vi "FXP NILIA_Shift_Arith.vi"(9 "dec":i32, 11 "x":i64) -> (3 "y":i64)   [LabVIEW 2012]
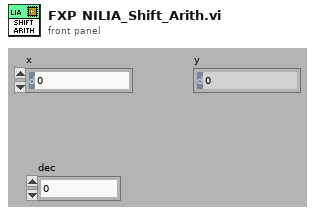
[diagram p1: front panel]
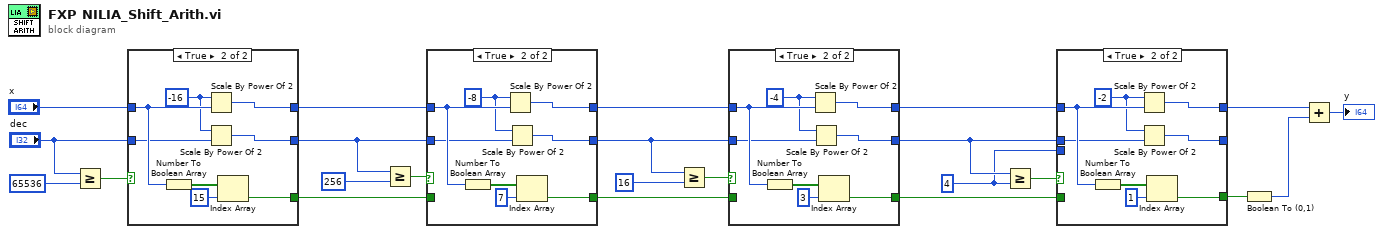
[diagram p0: block diagram]
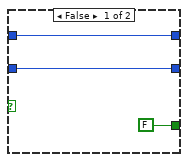
[diagram p5: hidden frame]
diagram:
  w8 = 4
  n1 = Greater Or Equal?(x="dec", y=65536) -> (x >= y?=w23:bool)
  n2 = case shown="True" w23 {
    tunnel: "x" -> [w26 w33]
    tunnel: [w26 w34] -> w16
    tunnel: "dec" -> [w25 w29]
    tunnel: [w25 w27] -> w19
    tunnel: [FALSE w30] -> w7
    frame False {
    }
    frame True {
      w28 = -16
      n3 = Number To Boolean Array(number=w33) -> (Boolean array=w32:bool[])
      n4 = Scale By Power Of 2(n=w28, x=w33) -> (x*2^n=w34:i64)
      n5 = Scale By Power Of 2(n=w28, x=w29) -> (x*2^n=w27:i32)
      n6 = Index Array(array=w32, index=15) -> (element=w30:bool)
    }
  }
  n7 = Greater Or Equal?(x=w19, y=256) -> (x >= y?=w18:bool)
  n8 = case shown="True" w18 {
    tunnel: w16 -> [w37 w44]
    tunnel: [w37 w45] -> w15
    tunnel: w19 -> [w36 w40]
    tunnel: [w36 w39] -> w13
    tunnel: w7 -> [w35 _]
    tunnel: [w35 w41] -> w6
    frame False {
    }
    frame True {
      w38 = -8
      n9 = Number To Boolean Array(number=w44) -> (Boolean array=w43:bool[])
      n10 = Scale By Power Of 2(n=w38, x=w44) -> (x*2^n=w45:i64)
      n11 = Scale By Power Of 2(n=w38, x=w40) -> (x*2^n=w39:i32)
      n12 = Index Array(array=w43, index=7) -> (element=w41:bool)
    }
  }
  n13 = Greater Or Equal?(x=w13, y=16) -> (x >= y?=w14:bool)
  n14 = case shown="True" w14 {
    tunnel: w15 -> [w48 w55]
    tunnel: [w48 w56] -> w11
    tunnel: w13 -> [w47 w51]
    tunnel: [w47 w50] -> w10
    tunnel: [w46 w52] -> w5
    tunnel: w6 -> [w46 _]
    frame False {
    }
    frame True {
      w49 = -4
      n15 = Number To Boolean Array(number=w55) -> (Boolean array=w54:bool[])
      n16 = Scale By Power Of 2(n=w49, x=w55) -> (x*2^n=w56:i64)
      n17 = Scale By Power Of 2(n=w49, x=w51) -> (x*2^n=w50:i32)
      n18 = Index Array(array=w54, index=3) -> (element=w52:bool)
    }
  }
  n19 = Greater Or Equal?(x=w10, y=w8) -> (x >= y?=w9:bool)
  n20 = case shown="True" w9 {
    tunnel: w11 -> [w59 w66]
    tunnel: [w59 w67] -> w4
    tunnel: w10 -> [w58 w62]
    tunnel: w8 -> [_ _]
    tunnel: [w58 w61] -> _
    tunnel: [w57 w63] -> w3
    tunnel: w5 -> [w57 _]
    frame False {
    }
    frame True {
      w60 = -2
      n21 = Number To Boolean Array(number=w66) -> (Boolean array=w65:bool[])
      n22 = Scale By Power Of 2(n=w60, x=w66) -> (x*2^n=w67:i64)
      n23 = Scale By Power Of 2(n=w60, x=w62) -> (x*2^n=w61:i32)
      n24 = Index Array(array=w65, index=1) -> (element=w63:bool)
    }
  }
  n25 = Boolean To (0,1)(Boolean=w3) -> (0, 1=w2:i16)
  n26 = Add(x=w4, y=w2) -> (x+y=→"y":i64)
